vi "Get XNET Signal Names.vi"(6 "Add Info?":bool, 7 "Parent Ref in":T1 format="%.0x", 8 "error in":errorcluster, 9 "Tree In":refnum<vi>, 10 "Parent":string, 11 "Frms":refnum<k21>[](array[refnum])) -> (0 "error out":errorcluster, 1 "Tree Out":refnum<vi>, 3 "XNET Signal Names":refnum<k21>[](array[refnum]))   [LabVIEW 2015, in "Protection and Counter Addon System Explorer.lvlib"]
uses:
  Protection and Counter Addon System Explorer.lvlib
  <vilib>/NI Veristand/Custom Device API/Custom Device Item Ref.ctl
  <vilib>/NI Veristand/Custom Device API/Custom Device Channel.ctl
  <vilib>/NI Veristand/Custom Device API/Custom Device Channel Type.ctl
  Shared/SubVIs/GUID Lookup.vi
  <vilib>/NI Veristand/Custom Device API/Set Item Property (U32).vi
  <resource>/objmgr/xnet.rc
  <vilib>/NI VeriStand/Custom Device API/Custom Device API.lvlib
  Shared/Protection and Counter Addon Shared.lvlib
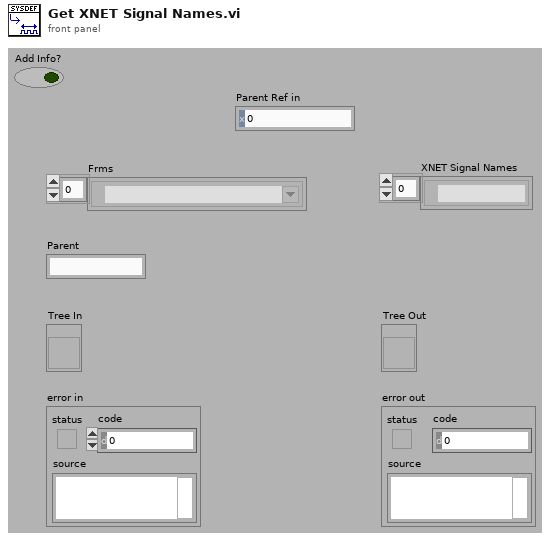
[diagram p1: front panel]
types:
  T1 = typedef "Custom Device API.lvlib/Custom Device Item Ref.ctl" = u64
  T2 = typedef "Custom Device API.lvlib/Custom Device Channel.ctl" = cluster{"Type":T3, "Units":string, "Default Value":dbl, "Faultable":bool, "Scalable":bool}
  T3 = typedef "Custom Device API.lvlib/Custom Device Channel Type.ctl" = enum16{"Input", "Output"}
  T4 = typedef "Custom Device API.lvlib/Custom Device Item Info.ctl" = cluster{"Name":string, "Is Channel":bool, "GUID":string, "Is Waveform":bool}
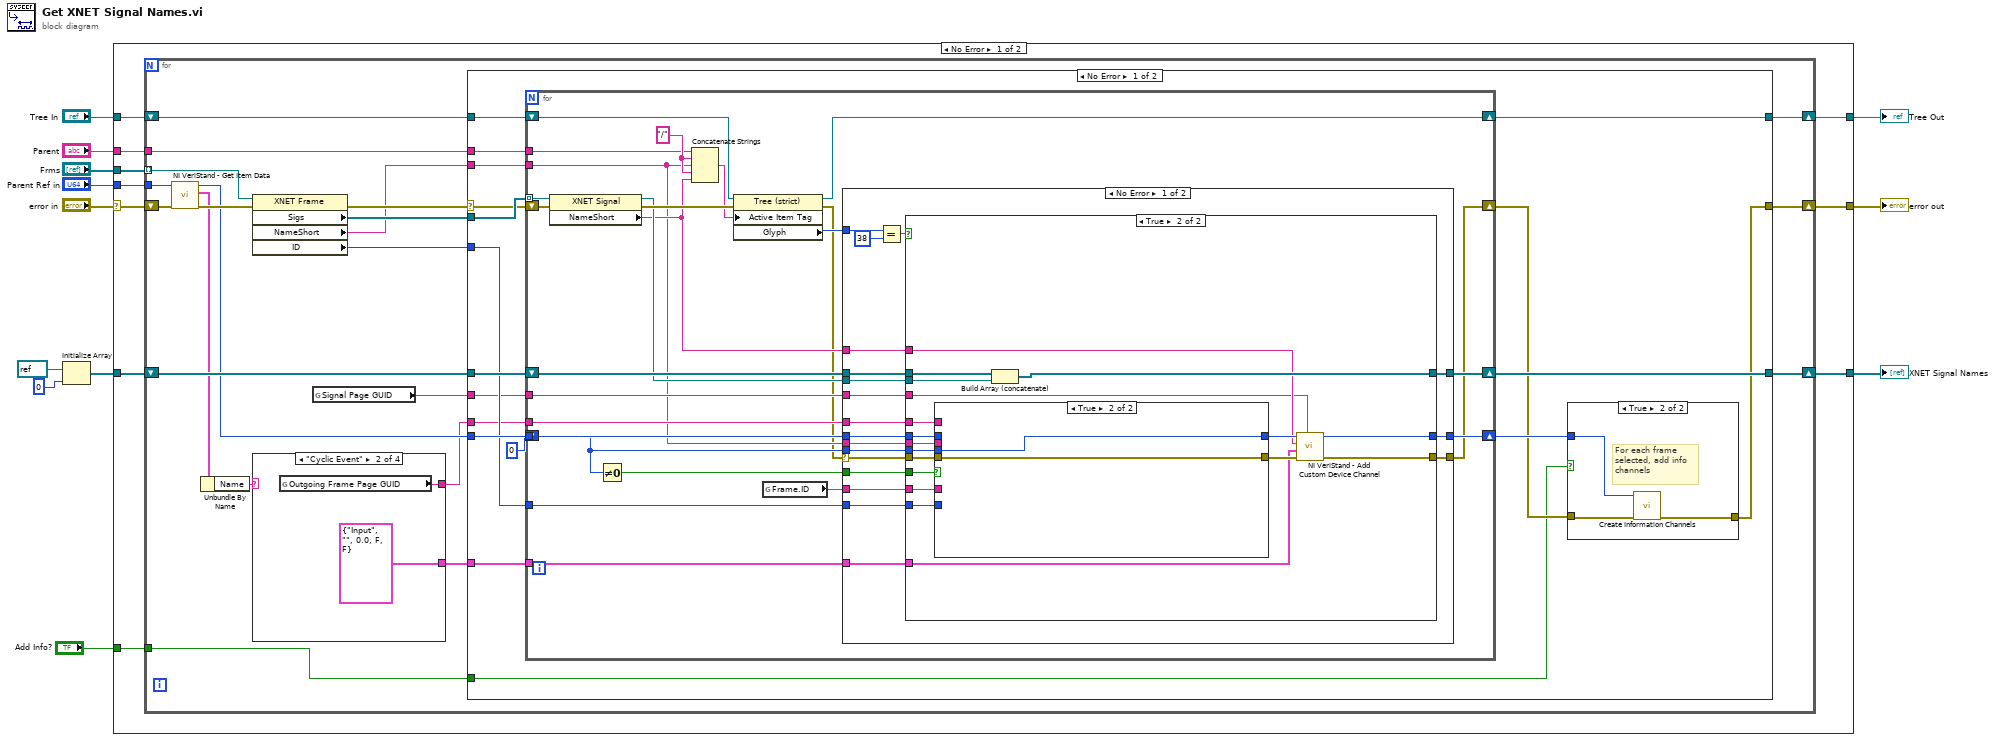
[diagram p0: block diagram]
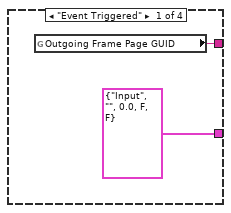
[diagram p2: hidden frame]
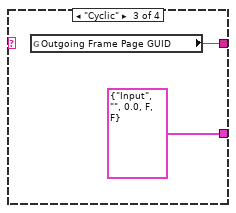
[diagram p3: hidden frame]
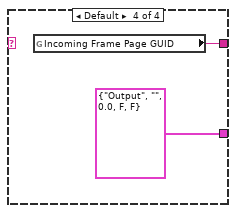
[diagram p4: hidden frame]
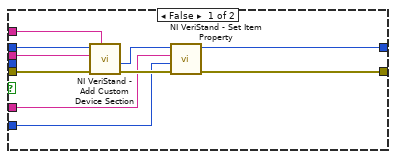
[diagram p7: hidden frame]
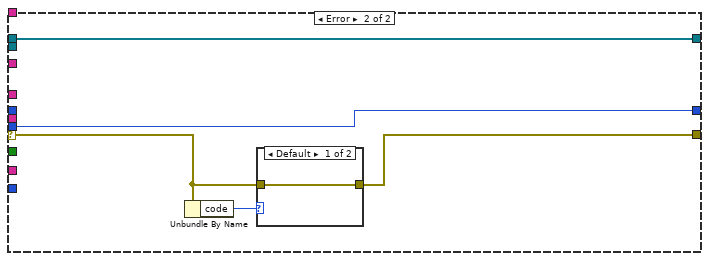
[diagram p8: hidden frame]
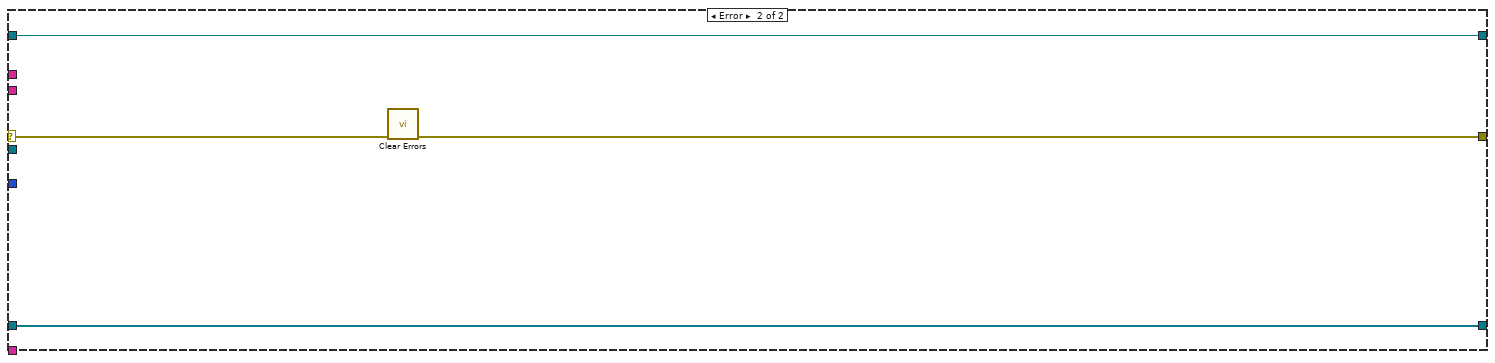
[diagram p10: hidden frame]
diagram:
  n1 = Initialize Array(refnum<k21> refnum ("XNET Signal"), 0 ("dimension size")) -> (w6:refnum<k21>[])
  n2 = case shown="No Error" "error in" {
    selector: "error in" -> [w19 w162]
    tunnel: "Parent" -> [w22 _]
    tunnel: [w21 w162] -> w11
    tunnel: "Frms" -> [w20 _]
    tunnel: [w18 _] -> w8
    tunnel: w6 -> [w17 _]
    tunnel: "Tree In" -> [w16 w161]
    tunnel: [w15 w161] -> w3
    tunnel: "Parent Ref in" -> [w14 _]
    tunnel: "Add Info?" -> [w13 _]
    frame No Error {
      n3 = for {
        shift-right: [w40] -> w21
        shift-left: w19 -> [w34]
        tunnel: w20 -> [w43] mode=indexing
        tunnel: w22 -> [w41]
        shift-right: [w37] -> w18
        shift-left: w17 -> [w38]
        shift-right: [w36] -> w15
        shift-left: w16 -> [w39]
        tunnel: w14 -> [w32]
        tunnel: w13 -> [w23]
        n4 = call <vilib>:"NI VeriStand - Get Item Data.vi"("error in (no error)"=w34, "Item Ref in"=w32) -> ("error out"=w33:errorcluster, "Item Info"=w30:T4, "Item Ref out"=w31:T1)  [unwired: 7 out]
        n5 = Unbundle By Name(w30) -> ("Name"=w29:string)
        n6 = property class="XNET Frame"(reference=w43, error in=w33) -> (error out=w35:errorcluster, "Sigs"=w42:refnum<k21>[], "NameShort"=w27:string, "ID"=w26:u32)  [unwired: 1 out]
        n7 = case shown="\"Cyclic Event\"" w29 {
          tunnel: [T2 {"Type"=enum."Input", "Units"="", "Default Value"=0.0, "Faultable"=FALSE, "Scalable"=FALSE} ("Channel") T2 {"Type"=enum."Input", "Units"="", "Default Value"=0.0, "Faultable"=FALSE, "Scalable"=FALSE} ("Channel") T2 {"Type"=enum."Input", "Units"="", "Default Value"=0.0, "Faultable"=FALSE, "Scalable"=FALSE} ("Channel") T2 {"Type"=enum."Output", "Units"="", "Default Value"=0.0, "Faultable"=FALSE, "Scalable"=FALSE} ("Channel")] -> w28
          tunnel: [w44 w46 w48 w50] -> w25
          frame "Event Triggered" {
            n8 = global read "GUID Lookup.vi" "Outgoing Frame Page GUID"() -> (w44:string)
          }
          frame "Cyclic Event" {
            n9 = global read "GUID Lookup.vi" "Outgoing Frame Page GUID"() -> (w46:string)
          }
          frame "Cyclic" {
            n10 = global read "GUID Lookup.vi" "Outgoing Frame Page GUID"() -> (w48:string)
          }
          frame Default {
            n11 = global read "GUID Lookup.vi" "Incoming Frame Page GUID"() -> (w50:string)
          }
        }
        n12 = global read "GUID Lookup.vi" "Signal Page GUID"() -> (w24:string)
        n13 = case shown="No Error" w35 {
          selector: w35 -> [w60 w157]
          tunnel: w42 -> [w69 _]
          tunnel: w27 -> [w68 _]
          tunnel: w41 -> [w67 _]
          tunnel: [w53 w158] -> w40
          tunnel: w39 -> [w66 w159]
          tunnel: w38 -> [w65 w160]
          tunnel: [w64 w160] -> w37
          tunnel: [w63 w159] -> w36
          tunnel: w31 -> [w62 _]
          tunnel: w26 -> [w59 _]
          tunnel: w24 -> [w58 _]
          tunnel: w25 -> [w57 _]
          tunnel: w28 -> [w56 _]
          tunnel: w23 -> [w52 _]
          frame No Error {
            n14 = for {
              tunnel: w69 -> [w98] mode=indexing
              tunnel: w68 -> [w77]
              tunnel: w67 -> [w95]
              shift-right: [w74] -> w54
              shift-left: w60 -> [w97]
              shift-right: [w90] -> w64
              shift-left: w65 -> [w89]
              shift-right: [w87] -> w63
              shift-left: w66 -> [w93]
              tunnel: w62 -> [w86]
              shift-right: [w85] -> w55
              shift-left: T1 0 ("Parent Ref out") -> [w84]
              tunnel: w59 -> [w81]
              tunnel: w58 -> [w80]
              tunnel: w57 -> [w79]
              tunnel: w56 -> [w78]
              w96 = "/" ("string")
              n15 = property class="XNET Signal"(reference=w98, error in=w97) -> (reference out=w88:refnum<k21>, error out=w94:errorcluster, "NameShort"=w82:string)
              n16 = Not Equal To 0?(x=w84) -> (x != 0?=w83:bool)
              n17 = Concatenate Strings(w95, w96, w77, w96, w82) -> (w92:string)
              n18 = property class="Tree (strict)"(reference=w93, error in=w94, "Active Item Tag"=w92) -> (reference out=w87:refnum<vi>, error out=w76:errorcluster, "Glyph"=w91:i32)
              n19 = global read "GUID Lookup.vi" "Frame.ID"() -> (w75:string)
              n20 = case shown="No Error" w76 {
                selector: w76 -> [w99 w152]
                tunnel: w91 -> [w117 _]
                tunnel: [w114 w154] -> w90
                tunnel: w89 -> [w113 w154]
                tunnel: w88 -> [w112 _]
                tunnel: [w111 w151] -> w74
                tunnel: w86 -> [w110 _]
                tunnel: [w109 w155] -> w85
                tunnel: w84 -> [w108 w155]
                tunnel: w83 -> [w107 _]
                tunnel: w82 -> [w106 _]
                tunnel: w81 -> [w105 _]
                tunnel: w75 -> [w104 _]
                tunnel: w80 -> [w103 _]
                tunnel: w79 -> [w102 _]
                tunnel: w78 -> [w101 _]
                tunnel: w77 -> [w100 _]
                frame No Error {
                  n21 = Equal?(x=w117, y=38) -> (x = y?=w115:bool)
                  n22 = case shown="True" w115 {
                    tunnel: [w120 w136] -> w114
                    tunnel: w113 -> [w120 w138]
                    tunnel: w112 -> [_ w137]
                    tunnel: w107 -> [_ w135]
                    tunnel: w100 -> [_ w134]
                    tunnel: w99 -> [w119 w133]
                    tunnel: [w119 w121] -> w111
                    tunnel: w110 -> [_ w132]
                    tunnel: [w118 w129] -> w109
                    tunnel: w108 -> [w118 w131]
                    tunnel: w106 -> [_ w127]
                    tunnel: w102 -> [_ w126]
                    tunnel: w103 -> [_ w125]
                    tunnel: w105 -> [_ w124]
                    tunnel: w104 -> [_ w123]
                    tunnel: w101 -> [_ w122]
                    frame False {
                    }
                    frame True {
                      n23 = case shown="True" w135 {
                        tunnel: w134 -> [w148 _]
                        tunnel: w133 -> [w147 w150]
                        tunnel: [w140 w150] -> w130
                        tunnel: w132 -> [w146 _]
                        tunnel: [w139 w149] -> w128
                        tunnel: w131 -> [_ w149]
                        tunnel: w126 -> [w145 _]
                        tunnel: w124 -> [w141 _]
                        tunnel: w123 -> [w142 _]
                        frame False {
                          n24 = call <vilib>:"NI VeriStand - Add Custom Device Section.vi"("GUID (Default Section)"=w145, "error in (no error)"=w147, "Section Name"=w148, "Parent Ref in"=w146) -> ("error out"=w143:errorcluster, "Section Ptr"=w144:T1)  [unwired: 4 in, 2 out]
                          n25 = call-poly <vilib>:"NI VeriStand - Set Item Property.vi"("error in (no error)"=w143, "Value"=w141, "Property Name"=w142, "Item Ref in"=w144) -> ("error out"=w140:errorcluster, "Item Ref out"=w139:T1)  [unwired: 5 in, 1 out]
                        }
                        frame True {
                        }
                      }
                      n26 = Build Array (concatenate)(w138, w137) -> (w136:refnum<k21>[])
                      n27 = call <vilib>:"NI VeriStand - Add Custom Device Channel.vi"("GUID (Default Channel)"=w125, "error in (no error)"=w130, "Channel"=w122, "Channel Name"=w127, "Parent Ref in"=w128) -> ("error out"=w121:errorcluster, "Parent Ref out"=w129:T1)  [unwired: 3 in, 2 out]
                    }
                  }
                }
                frame Error {
                  n28 = Unbundle By Name(w152) -> ("code"=w153:i32)
                  n29 = case shown="Default" w153 {
                    tunnel: [w156 _] -> w151
                    tunnel: w152 -> [w156 _]
                    frame Default {
                    }
                    frame 1136 {
                    }
                  }
                }
              }
            }
            n30 = case shown="True" w52 {
              tunnel: w55 -> [_ w73]
              tunnel: w54 -> [w70 w72]
              tunnel: [w70 w71] -> w53
              frame False {
              }
              frame True {
                # "For each frame \nselected, add info\nchannels"
                n31 = call "Create Information Channels.vi"("error in (no error)"=w72, "Node Ptr"=w73) -> ("error out"=w71:errorcluster)  [unwired: 8 in]
              }
            }
          }
          frame Error {
            n32 = call <vilib>:"Clear Errors.vi"("error in (no error)"=w157) -> ("error out"=w158:errorcluster)  [unwired: 5 in, 1 out]
          }
        }
      }
    }
    frame Error {
    }
  }
  "error out" <- w11
  "XNET Signal Names" <- w8
  "Tree Out" <- w3
